vi "ENPH 354 Assignment 1 - Q5.vi"() -> ()   [LabVIEW 2021]
panel:
  out "Numeric":dbl
  out "x > y?":bool
  out "String":string
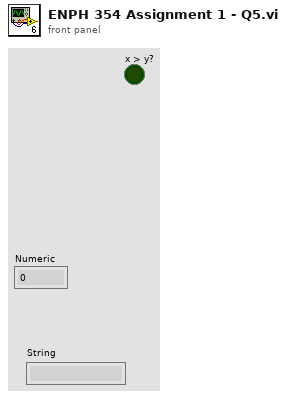
[diagram p1: front panel]
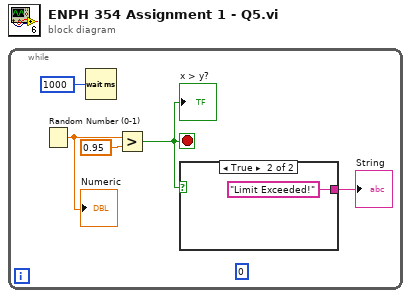
[diagram p0: block diagram]
diagram:
  n1 = while {
    stop <- w3 stop-if-true
    (unwired) u32 0 ("millisecond timer value")
    n2 = Random Number (0-1)() -> (number: 0 to 1=w1:dbl)
    "Numeric" <- w1
    n3 = Wait (ms)(milliseconds to wait=u32 1000) -> ()  [unwired: 1 out]
    n4 = Greater?(x=w1, y=0.95) -> (0:w3:bool)
    "x > y?" <- w3
    n5 = case shown="True" w3 {
      tunnel: [_ "Limit Exceeded!" ("String")] -> w2
      frame False {
      }
      frame True {
      }
    }
    "String" <- w2
  }
